vi "VisualizeSamp.vi"() -> ()   [LabVIEW 2014, in "Visualization.lvlib" / "VisualizeSamp.lvclass"]
uses:
  VisualizeSamp.lvclass
  VisualizeBase/VisualizeBase_class/Requests/clUserEventType.ctl
  <vilib>/event_ctls.llb/usereventprio.ctl
  <vilib>/Utility/error.llb/Error Cluster From Error Code.vi
  <vilib>/ErrorRing/Error Ring.xnode
  VisualizeBase/VisualizeBase_class/VisualizeBase.lvclass
  <userlib>/NIST/NISTErrorLib/NISTErrorLib.lvlib
  Digitizer/DigitizerModule/DigitizerModule.lvlib
panel:
  in  "btnReset":bool
  in  "btnClear":bool
  in  "Concatenate Inputs":bool
  out "Current Samples":dbl[][](graph)
  out "Voltage Samples":dbl[][](graph)
  in  "QueName":string="VisSamples"
  out "ErrorArray":errorcluster[](array[cluster])
  in  "btnStop":bool
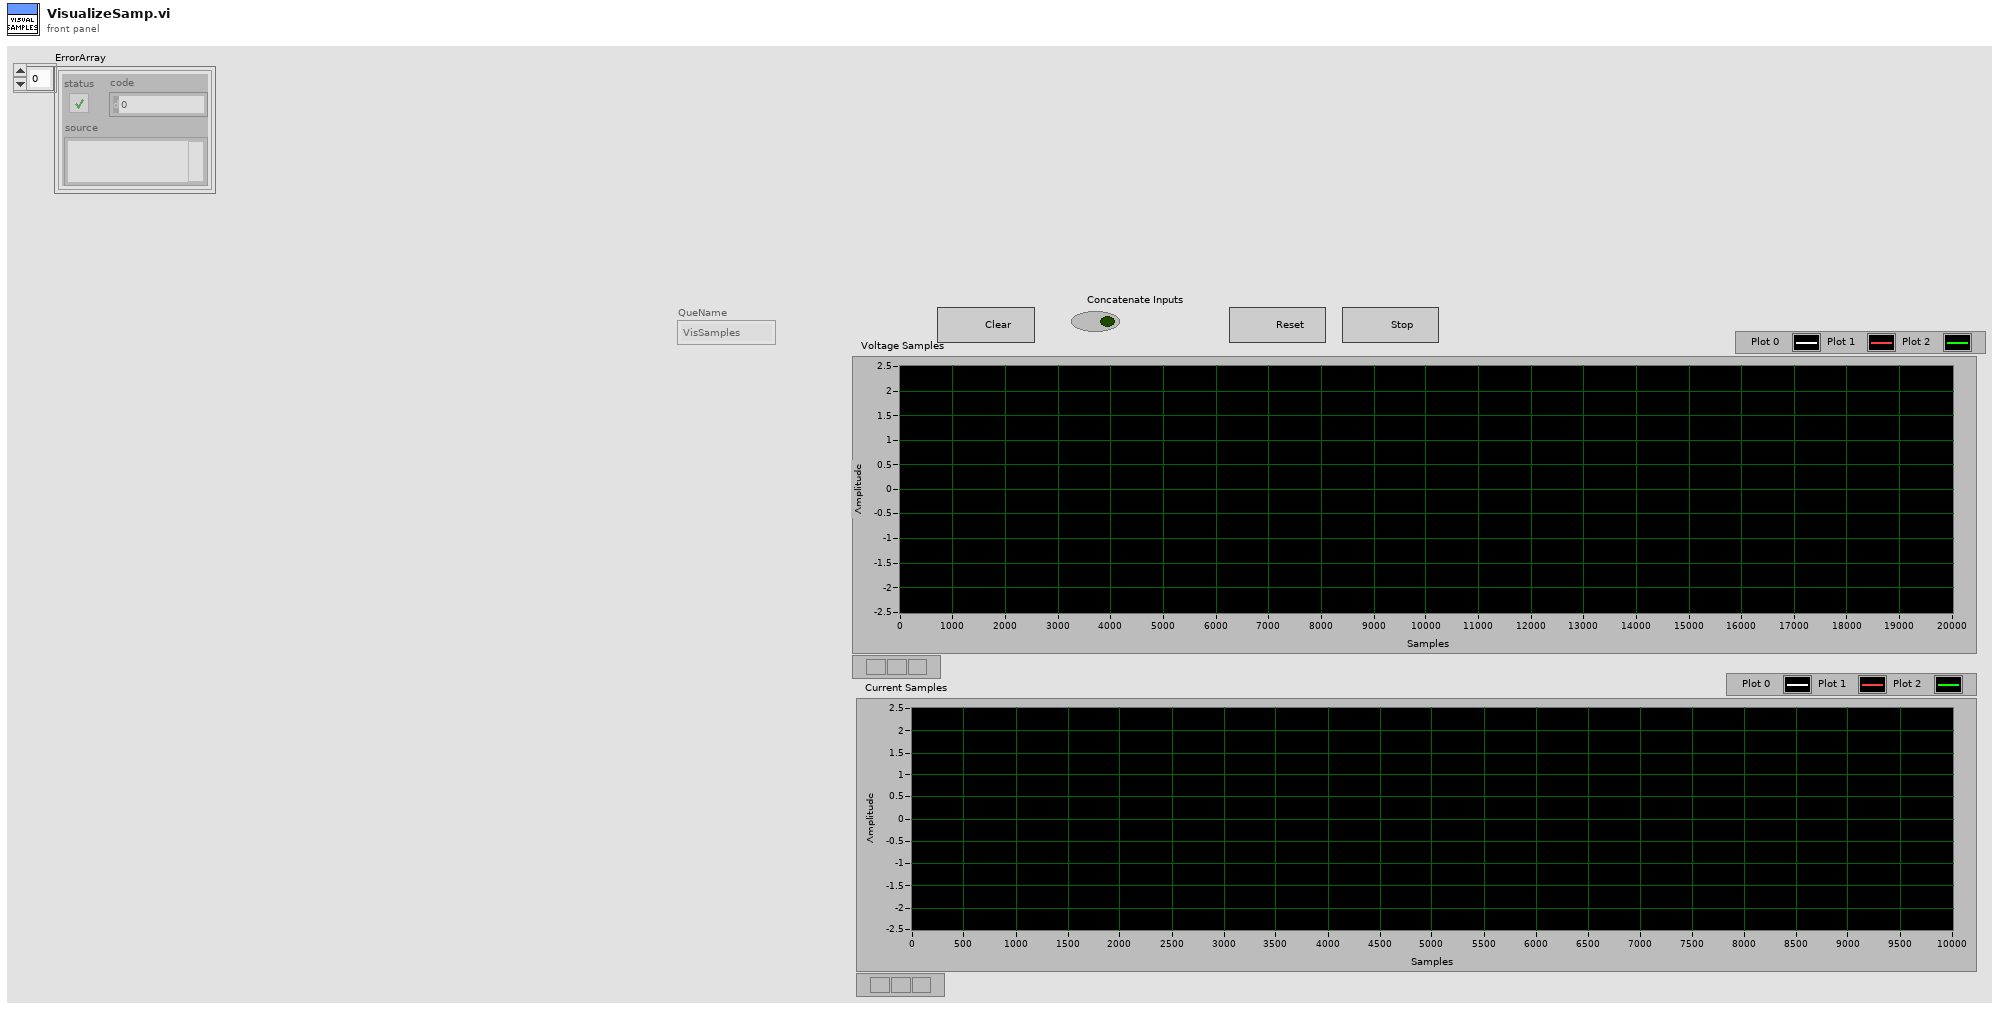
[diagram p1: front panel]
types:
  T1 = typedef "Visualization.lvlib/VisualizeBase.lvclass/clRequestEvents.ctl" = cluster{"StopRequest":refnum<user-event>, "ResetRequest":refnum<user-event>}
  T2 = typedef "DigitizerModule.lvlib/clBroadcastEvents.ctl" = cluster{"DidInit":refnum<user-event>, "StatusUpdate":refnum<user-event>, "ErrorReport":refnum<user-event>, "DidStop":refnum<user-event>, "PathToINI":refnum<user-event>, "Channels":refnum<user-event>, "Acq":refnum<user-event>, "Trigger":refnum<user-event>, "Waveforms":refnum<user-event>}
  T3 = typedef "Visualization.lvlib/VisualizeBase.lvclass/clUserEventType.ctl" = cluster{"BusIndex":i8, "Data":variant}
  T4 = typedef "usereventprio.ctl" = enum32{"high priority", "normal priority"}
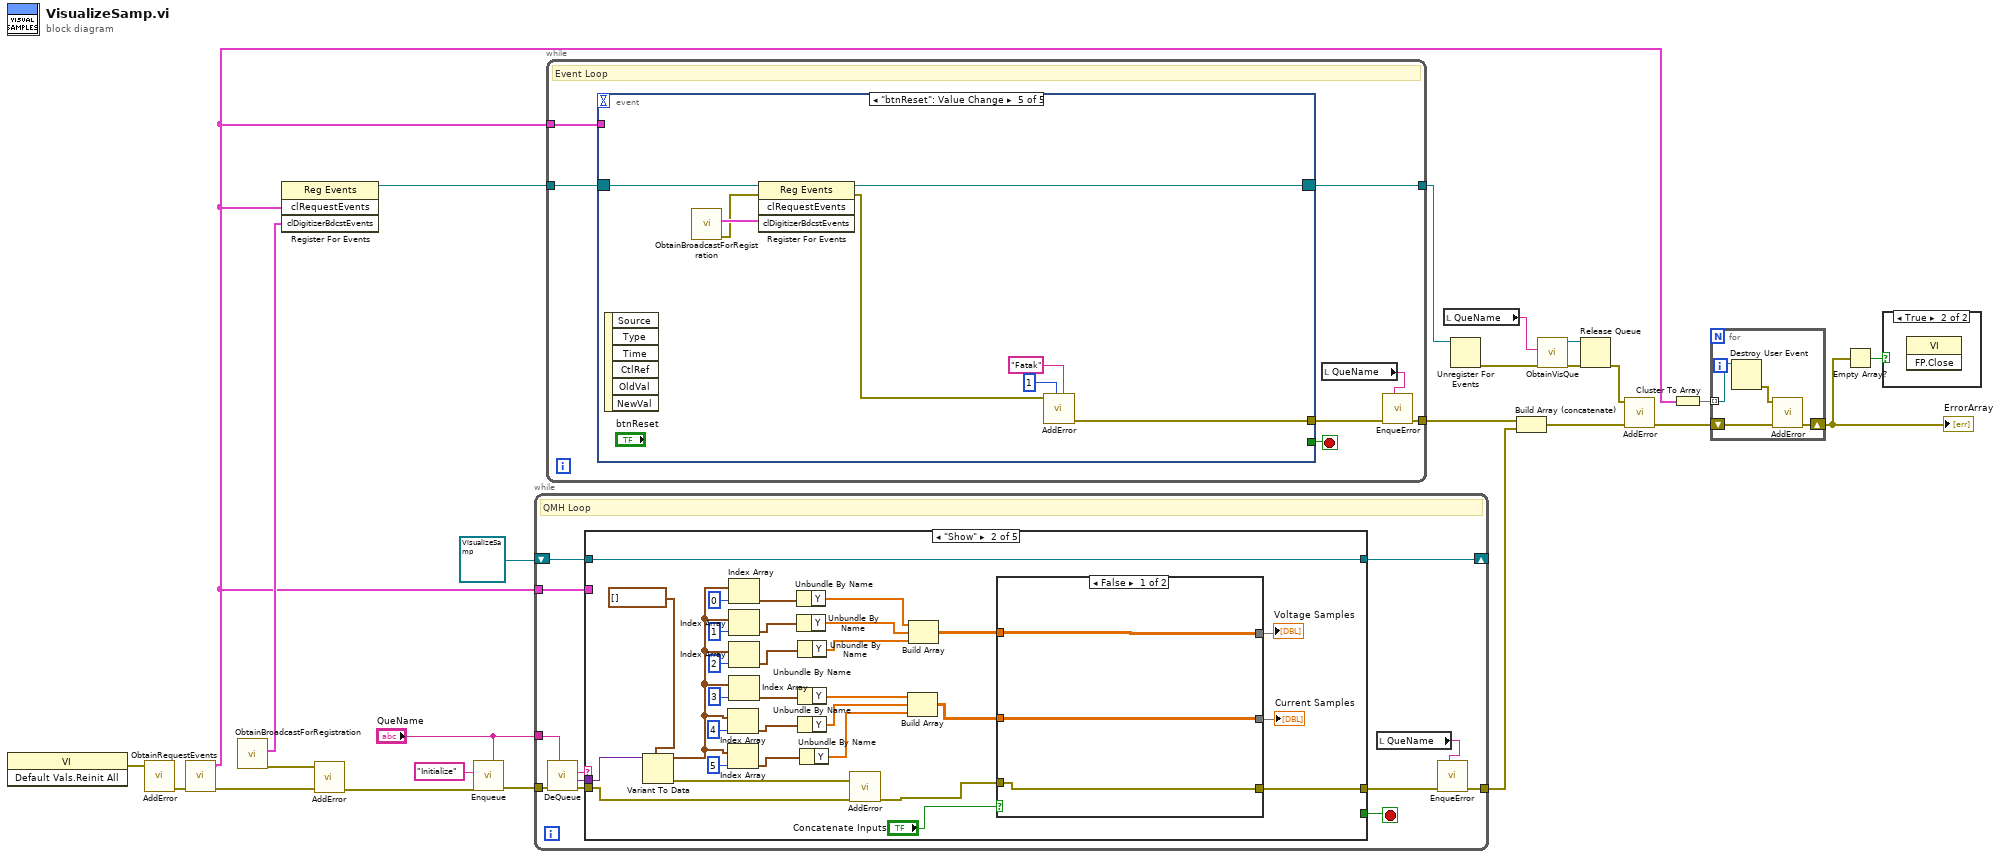
[diagram p0: block diagram]
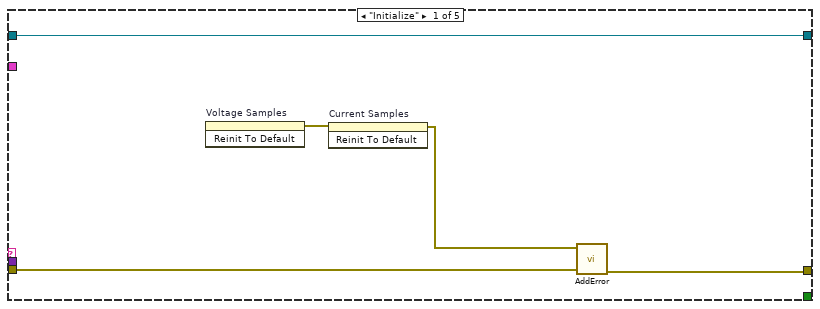
[diagram p3: hidden frame]
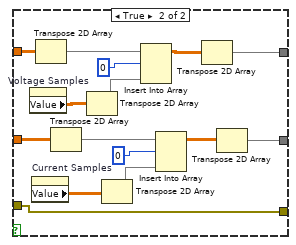
[diagram p4: hidden frame]
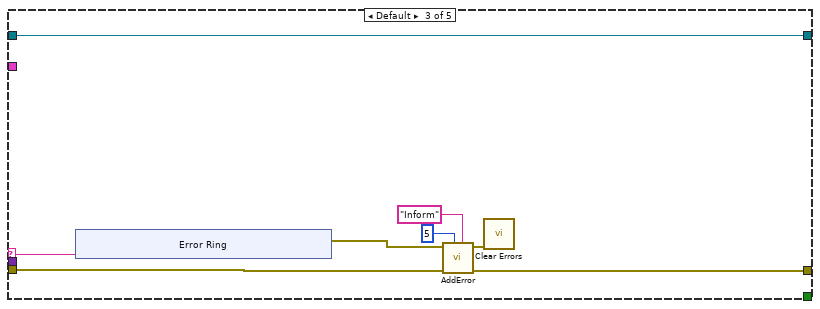
[diagram p5: hidden frame]
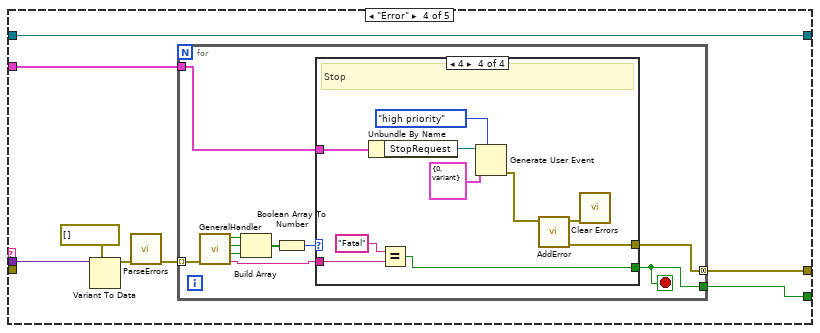
[diagram p6: hidden frame]
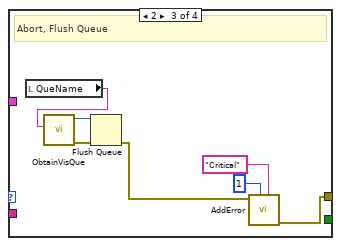
[diagram p9: hidden frame]
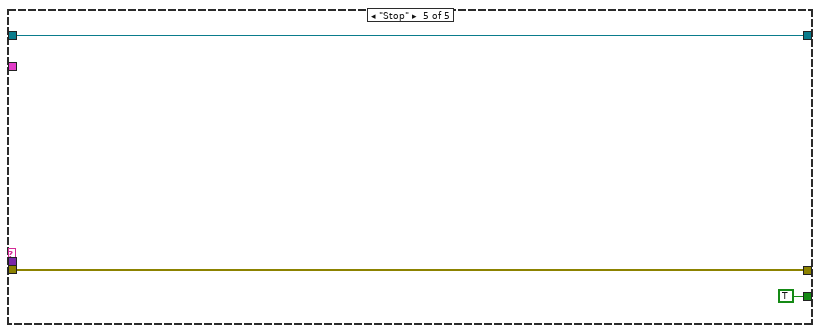
[diagram p10: hidden frame]
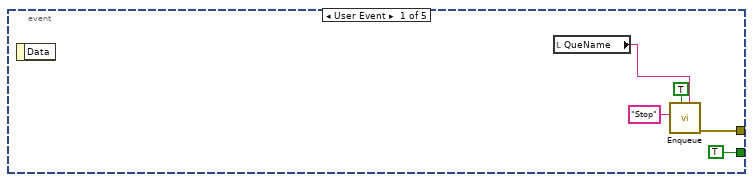
[diagram p11: hidden frame]
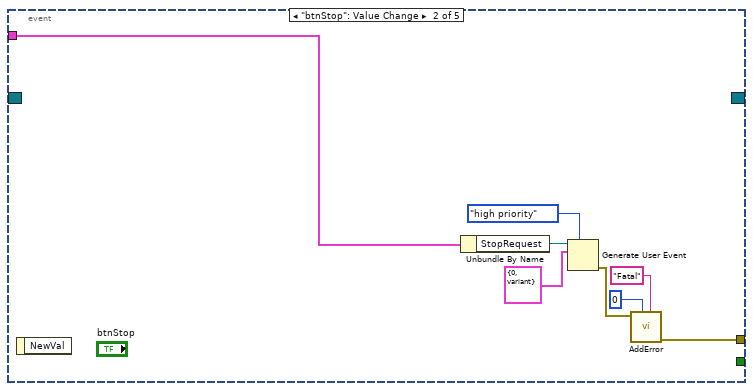
[diagram p12: hidden frame]
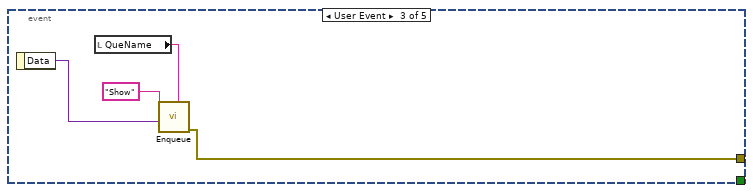
[diagram p13: hidden frame]
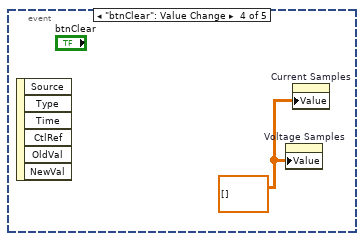
[diagram p14: hidden frame]
diagram:
  n1 = invoke class="VI" method="Default Vals.Reinit All"() -> (error out=w20:errorcluster)  [unwired: 3 in, 2 out]
  n2 = call <userlib>:"AddError.vi"("error in (no error)"=w20) -> ("ErrorArray"=w19:errorcluster[])  [unwired: 9 in, 1 out]
  n3 = call "ObtainRequestEvents.vi"("Error"=w19) -> ("Error"=w16:errorcluster[], "clRequestEvents"=w1:T1)  [unwired: 9 in]
  n4 = call "ObtainBroadcastForRegistration.vi"() -> ("error out"=w17:errorcluster, "clDigitizerBdcstEvents"=w13:T2)  [unwired: 10 in]
  n5 = register-events(w1, w13) -> (reference out=w23:refnum<event-registration>)  [unwired: 2 in, 1 out]
  n6 = call <userlib>:"AddError.vi"("ErrorArray"=w16, "error in (no error)"=w17) -> ("ErrorArray"=w15:errorcluster[])  [unwired: 8 in, 1 out]
  n7 = call "Enqueue.vi"("QueName"="QueName", "Error"=w15, "Message"="Initialize") -> ("Error"=w24:errorcluster[])  [unwired: 8 in]
  n8 = while {
    tunnel: w24 -> [w37]
    tunnel: [w31] -> w22
    tunnel: "QueName" -> [w29]
    shift-right: [w28] -> _
    shift-left: refnum<class "VisualizeSamp.lvclass"> refnum ("VisualizeBase_class.lvclass") -> [w27]
    tunnel: w1 -> [w26]
    stop <- w32 stop-if-true
    # "QMH Loop"
    n9 = call "DeQueue.vi"("QueName"=w29, "Error"=w37) -> ("Error"=w34:errorcluster[], "Data"=w35:variant, "Message"=w36:string)  [unwired: 7 in]
    n10 = case shown="\"Show\"" w36 {
      selector: w36 -> [_ _ w99 _ _]
      tunnel: w35 -> [_ w72 _ w114 _]
      tunnel: w34 -> [w39 w71 w97 _ w143]
      tunnel: [w40 w59 w96 w110 w143] -> w33
      tunnel: [_ _ _ w109 TRUE] -> w32
      tunnel: w27 -> [w42 w73 w92 w108 w142]
      tunnel: [w42 w73 w92 w108 w142] -> w28
      tunnel: w26 -> [_ _ _ w107 _]
      frame "Initialize" {
        n11 = invoke on="Voltage Samples" class="WFGraph (strict)" method="Reinit To Default"() -> (error out=w41:errorcluster)  [unwired: 3 in, 2 out]
        n12 = invoke on="Current Samples" class="WFGraph (strict)" method="Reinit To Default"(error in=w41) -> (error out=w38:errorcluster)  [unwired: 2 in, 2 out]
        n13 = call <userlib>:"AddError.vi"("ErrorArray"=w39, "error in (no error)"=w38) -> ("ErrorArray"=w40:errorcluster[])  [unwired: 8 in, 1 out]
      }
      frame "Show" {
        n14 = Variant To Data(type=waveform(dbl)[] [], Variant=w72) -> (data=w63:waveform(dbl)[], error out=w70:errorcluster)  [unwired: 1 in]
        n15 = Index Array(array=w63, index=4) -> (element=w47:waveform(dbl))
        n16 = Index Array(array=w63, index=5) -> (element=w46:waveform(dbl))
        n17 = Index Array(array=w63, index=0) -> (element=w54:waveform(dbl))
        n18 = Index Array(array=w63, index=1) -> (element=w52:waveform(dbl))
        n19 = Index Array(array=w63, index=2) -> (element=w50:waveform(dbl))
        n20 = Index Array(array=w63, index=3) -> (element=w48:waveform(dbl))
        n21 = Unbundle By Name(w54) -> ("Y"=w53:dbl[])
        n22 = Unbundle By Name(w52) -> ("Y"=w51:dbl[])
        n23 = Unbundle By Name(w50) -> ("Y"=w49:dbl[])
        n24 = Unbundle By Name(w48) -> ("Y"=w45:dbl[])
        n25 = Unbundle By Name(w47) -> ("Y"=w44:dbl[])
        n26 = Unbundle By Name(w46) -> ("Y"=w43:dbl[])
        n27 = call <userlib>:"AddError.vi"("ErrorArray"=w71, "error in (no error)"=w70) -> ("ErrorArray"=w60:errorcluster[])  [unwired: 8 in, 1 out]
        n28 = Build Array(w45, w44, w43) -> (w57:dbl[][])
        n29 = Build Array(w53, w51, w49) -> (w58:dbl[][])
        n30 = case shown="False" "Concatenate Inputs" {
          tunnel: w58 -> [w75 w88]
          tunnel: [w75 w86] -> w62
          tunnel: w60 -> [w76 w91]
          tunnel: [w76 w91] -> w59
          tunnel: w57 -> [w74 w79]
          tunnel: [w74 w80] -> w56
          frame False {
          }
          frame True {
            n31 = property on="Voltage Samples" class="WFGraph (strict)"() -> ("Value"=w89:dbl[][])  [unwired: 2 in, 2 out]
            n32 = property on="Current Samples" class="WFGraph (strict)"() -> ("Value"=w81:dbl[][])  [unwired: 2 in, 2 out]
            n33 = Transpose 2D Array(2D array=w88) -> (transposed array=w85:dbl[][])
            n34 = Transpose 2D Array(2D array=w79) -> (transposed array=w78:dbl[][])
            n35 = Transpose 2D Array(2D array=w89) -> (transposed array=w84:dbl[][])
            n36 = Transpose 2D Array(2D array=w81) -> (transposed array=w83:dbl[][])
            n37 = Insert Into Array(array=w85, index (row)=0, new element=w84) -> (w90:dbl[][])  [unwired: 1 in]
            n38 = Insert Into Array(array=w78, index (row)=0, new element=w83) -> (w77:dbl[][])  [unwired: 1 in]
            n39 = Transpose 2D Array(2D array=w90) -> (transposed array=w86:dbl[][])
            n40 = Transpose 2D Array(2D array=w77) -> (transposed array=w80:dbl[][])
          }
        }
        "Voltage Samples" <- w62
        "Current Samples" <- w56
      }
      frame Default {
        n41 = xnode "Error Ring"("parameter 0"=w99) -> ("error out"=w98:errorcluster)
        n42 = call <userlib>:"AddError.vi"("Severity"="Inform" ("String"), "Priority"=u8 5, "ErrorArray"=w97, "error in (no error)"=w98) -> ("ErrorArray"=w96:errorcluster[], "error out"=w95:errorcluster)  [unwired: 6 in]
        n43 = call <vilib>:"Clear Errors.vi"("error in (no error)"=w95) -> ()  [unwired: 5 in, 2 out]
      }
      frame "Error" {
        n44 = Variant To Data(type=errorcluster[] [], Variant=w114) -> (data=w112:errorcluster[])  [unwired: 1 in, 1 out]
        n45 = call <userlib>:"ParseErrors.vi"("ErrorArray"=w112) -> ("ErrorArray"=w111:errorcluster[])  [unwired: 8 in, 2 out]
        n46 = for {
          tunnel: w111 -> [w124] mode=indexing
          tunnel: [w118] -> w110 mode=concatenating
          tunnel: [w116] -> w109
          tunnel: w107 -> [w115]
          stop <- w116 stop-if-true
          n47 = call <userlib>:"GeneralHandler.vi"("error in (no error)"=w124) -> ("Severity"=w117:string, "Stop"=w121:bool, "Abort"=w122:bool, "Continue"=w123:bool)  [unwired: 7 in]
          n48 = Build Array(w123, w122, w121) -> (w120:bool[])
          n49 = Boolean Array To Number(Boolean array=w120) -> (number=w119:u32)
          n50 = case shown="4" w119 {
            tunnel: [_ _ w129 w140] -> w118
            tunnel: w117 -> [_ _ _ w135]
            tunnel: [_ _ _ w133] -> w116
            tunnel: w115 -> [_ _ _ w132]
            frame 0, Default {
              # "No Dialog"
            }
            frame 1 {
              # "Continue"
            }
            frame 2 {
              # "Abort, Flush Queue"
              n51 = local read "QueName"() -> (w125:string)
              n52 = call "ObtainVisQue.vi"("QueName"=w125) -> ("error out"=w131:errorcluster, "queue out"=w130:refnum<queue>)  [unwired: 9 in]
              n53 = Flush Queue(queue=w130, error in (no error)=w131) -> (error out=w128:errorcluster)  [unwired: 2 out]
              n54 = call <userlib>:"AddError.vi"("Severity"="Critical" ("String"), "Priority"=u8 1, "error in (no error)"=w128) -> ("ErrorArray"=w129:errorcluster[])  [unwired: 7 in, 1 out]
            }
            frame 4 {
              # "Stop"
              n55 = Unbundle By Name(w132) -> ("StopRequest"=w141:refnum<user-event>)
              n56 = Equal?(x="Fatal", y=w135) -> (x = y?=w133:bool)
              n57 = Generate User Event(priority (normal)=usereventprio."high priority", user event=w141, event data cluster=T3 {"BusIndex"=0, "Data"=variant} ("event data")) -> (error out=w139:errorcluster)  [unwired: 1 in, 1 out]
              n58 = call <userlib>:"AddError.vi"("error in (no error)"=w139) -> ("ErrorArray"=w140:errorcluster[], "error out"=w136:errorcluster)  [unwired: 9 in]
              n59 = call <vilib>:"Clear Errors.vi"("error in (no error)"=w136) -> ()  [unwired: 5 in, 2 out]
            }
          }
        }
      }
      frame "Stop" {
      }
    }
    n60 = local read "QueName"() -> (w30:string)
    n61 = call "EnqueError.vi"("QueName"=w30, "Error"=w33) -> ("Error"=w31:errorcluster[])  [unwired: 9 in]
  }
  n62 = while {
    tunnel: w23 -> [w151]
    tunnel: [w148] -> w21
    tunnel: w1 -> [w146]
    tunnel: [w145] -> w12
    stop <- w150 stop-if-true
    # "Event Loop"
    n63 = event shown="[4] \"btnReset\": Value Change" {
      selector: w151 -> [_ _ _ _ w177]
      dyn-events: [_ _ _ _ w170] -> w145
      timeout: _ -> [_ _ _ _ _]
      tunnel: [TRUE _ _ _ _] -> w150
      tunnel: [w155 w162 w166 _ w174] -> w149
      tunnel: w146 -> [_ w157 _ _ _]
      event User Event {
        n64 = event-data() -> ()  [unwired: 1 in, 1 out]
        n65 = local read "QueName"() -> (w152:string)
        n66 = call "Enqueue.vi"("QueName"=w152, "Priority? (F)"=TRUE, "Message"="Stop") -> ("Error"=w155:errorcluster[])  [unwired: 8 in]
      }
      event "btnStop": Value Change {
        n67 = event-data() -> ()  [unwired: 1 in, 1 out]
        n68 = Unbundle By Name(w157) -> ("StopRequest"=w163:refnum<user-event>)
        n69 = Generate User Event(priority (normal)=usereventprio."high priority", user event=w163, event data cluster=T3 {"BusIndex"=0, "Data"=variant} ("event data")) -> (error out=w164:errorcluster)  [unwired: 1 in, 1 out]
        n70 = call <userlib>:"AddError.vi"("Severity"="Fatal" ("String"), "Priority"=u8 0, "error in (no error)"=w164) -> ("ErrorArray"=w162:errorcluster[])  [unwired: 7 in, 1 out]
      }
      event User Event {
        n71 = event-data() -> ("Data"=w167:variant)  [unwired: 1 in]
        n72 = local read "QueName"() -> (w165:string)
        n73 = call "Enqueue.vi"("QueName"=w165, "Data"=w167, "Message"="Show") -> ("Error"=w166:errorcluster[])  [unwired: 8 in]
      }
      event "btnClear": Value Change {
        w169 = dbl[][] [] ("Voltage Samples")
        n74 = event-data() -> ()  [unwired: 1 in, 6 out]
        n75 = property on="Voltage Samples" class="WFGraph (strict)"("Value"=w169) -> ()  [unwired: 2 in, 2 out]
        n76 = property on="Current Samples" class="WFGraph (strict)"("Value"=w169) -> ()  [unwired: 2 in, 2 out]
      }
      event "btnReset": Value Change {
        n77 = event-data() -> ()  [unwired: 1 in, 6 out]
        n78 = call "ObtainBroadcastForRegistration.vi"() -> ("error out"=w175:errorcluster, "clDigitizerBdcstEvents"=w176:T2)  [unwired: 10 in]
        n79 = register-events(reference=w177, error in=w175, w176) -> (reference out=w170:refnum<event-registration>, error out=w173:errorcluster)  [unwired: 1 in]
        n80 = call <userlib>:"AddError.vi"("Severity"="Fatak", "Priority"=u8 1, "error in (no error)"=w173) -> ("ErrorArray"=w174:errorcluster[])  [unwired: 7 in, 1 out]
      }
    }
    n81 = local read "QueName"() -> (w147:string)
    n82 = call "EnqueError.vi"("QueName"=w147, "Error"=w149) -> ("Error"=w148:errorcluster[])  [unwired: 9 in]
  }
  n83 = local read "QueName"() -> (w11:string)
  n84 = Unregister For Events(event registration refnum=w12) -> (error out=w10:errorcluster)  [unwired: 1 in]
  n85 = Build Array (concatenate)(w21, w22) -> (w6:errorcluster[])
  n86 = call "ObtainVisQue.vi"("error in (no error)"=w10, "QueName"=w11) -> ("error out"=w8:errorcluster, "queue out"=w9:refnum<queue>)  [unwired: 8 in]
  n87 = Release Queue(queue=w9, error in (no error)=w8) -> (error out=w7:errorcluster)  [unwired: 1 in, 2 out]
  n88 = call <userlib>:"AddError.vi"("ErrorArray"=w6, "error in (no error)"=w7) -> ("ErrorArray"=w5:errorcluster[])  [unwired: 8 in, 1 out]
  n89 = Cluster To Array(cluster=w1) -> (array=w4:refnum<user-event>[])
  n90 = for {
    tunnel: w4 -> [w181] mode=indexing
    shift-right: [w180] -> w2
    shift-left: w5 -> [w179]
    n91 = Destroy User Event(user event=w181) -> (error out=w178:errorcluster)  [unwired: 1 in]
    n92 = call <userlib>:"AddError.vi"("ErrorArray"=w179, "error in (no error)"=w178) -> ("ErrorArray"=w180:errorcluster[])  [unwired: 8 in, 1 out]
  }
  "ErrorArray" <- w2
  n93 = Empty Array?(array=w2) -> (empty?=w3:bool)
  n94 = case shown="True" w3 {
    frame False {
    }
    frame True {
      n95 = invoke class="VI" method="FP.Close"() -> ()  [unwired: 3 in, 3 out]
    }
  }
